vi "serial_monitor.vi"(1 "ON\nOFF":bool=TRUE caption="Init", 2 "Porta seriale":refnum<visa-resource-name>="COM3") -> ()   [LabVIEW 2014]
doc: "Lettura continua da porta seriale , INIT (true or false) della porta (9600, & bit, 1stop bit, EVEN)\nSalva su file\nFM&ADL aprile 2012"
uses:
  <vilib>/Instr/_visa.llb/VISA Configure Serial Port (Instr).vi
panel:
  out "error out":errorcluster
  out "Tutti i dati":string="MAGNETOMETRO\r\nversione Luglio 2015\r\nInizio esecuzione\r\nC9A1 D486 D53\r\n-1.69910 -1.35864 0.41638\r\n C95B D4AE D56\r\n-1.70764 -1.35376 0.41675\r\n C9AF D486 D41\r\n-1.69739 -1.35864 0.41418\r\n C997 D4B4 CED\r\n-1.70032 -1.35303 0.40393\r\n "
  in  "Baud rate":u32(ring)=9600 items=["9600"=9600, "14400"=14400, "19200"=19200, "38400"=38400, "57600"=57600, "115200"=115200]
  in  "SALVA I DATI SU FILE":bool=TRUE caption="ON\nOFF"
  out "Dati":i32[](graph)
  out "N_dati":u32
  out "lung":i32
  in  "stop":bool
  out "Number of Bytes at Serial Port":u32
  out "Dati trasmessi":string
  # "NO\nSI"
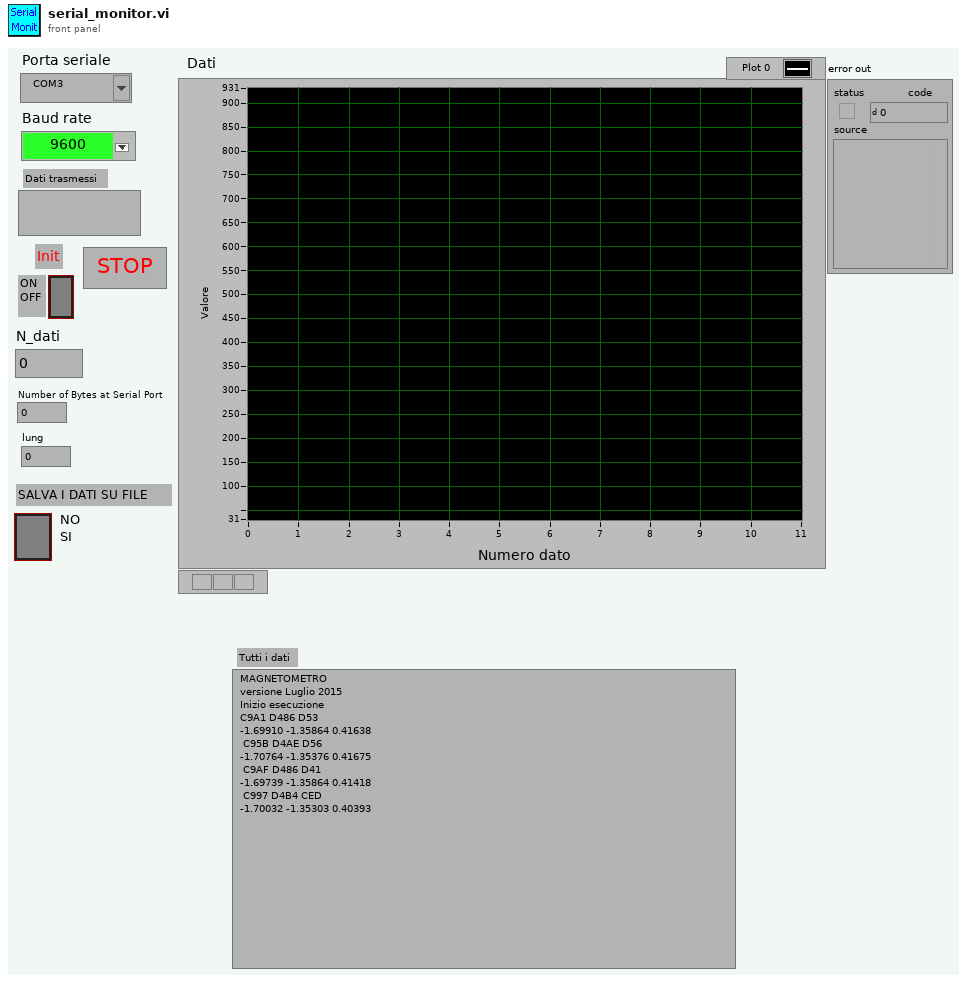
[diagram p1: front panel]
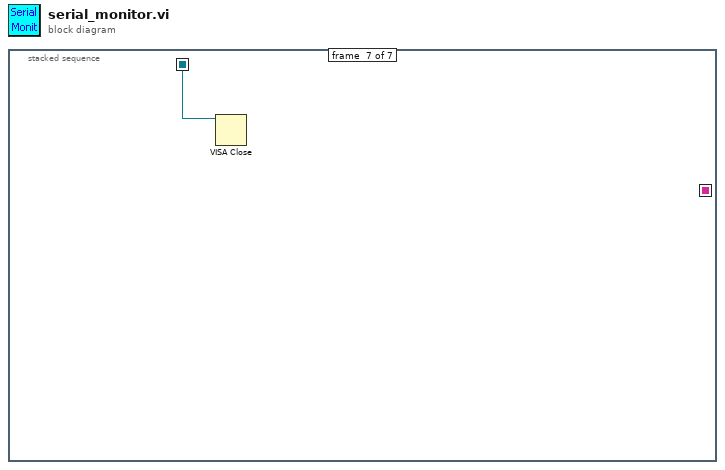
[diagram p0: block diagram]
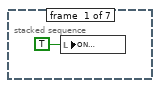
[diagram p2: hidden frame]
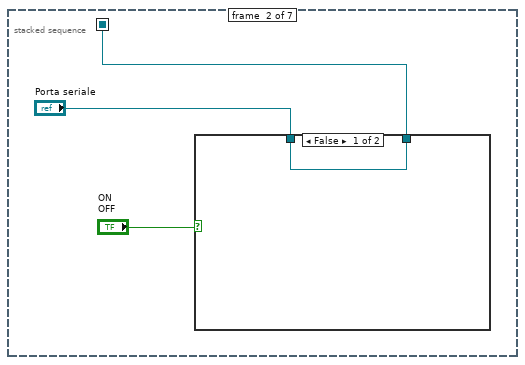
[diagram p3: hidden frame]
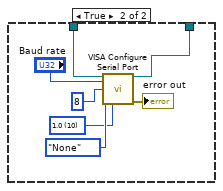
[diagram p4: hidden frame]
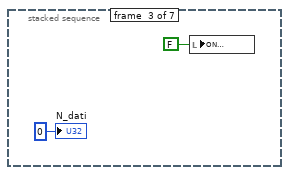
[diagram p5: hidden frame]
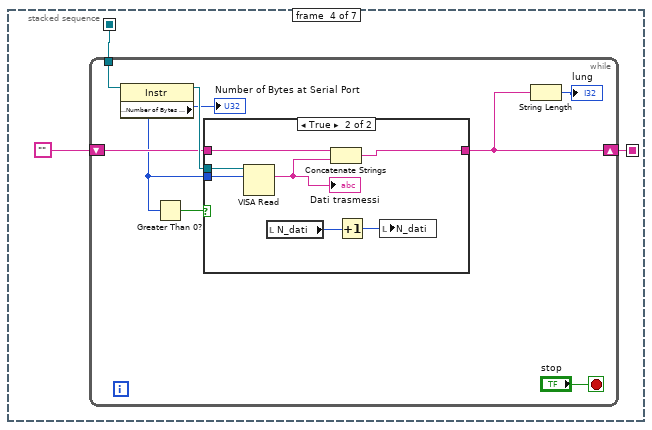
[diagram p6: hidden frame]
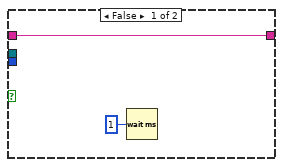
[diagram p7: hidden frame]
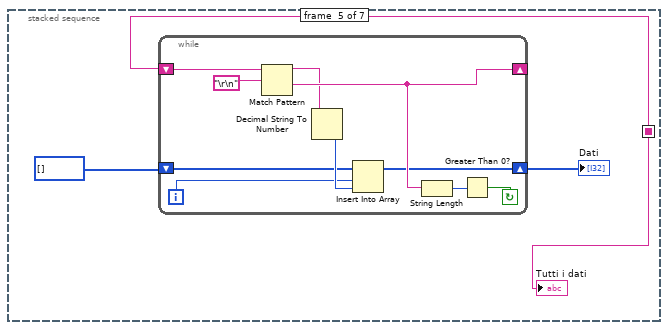
[diagram p8: hidden frame]
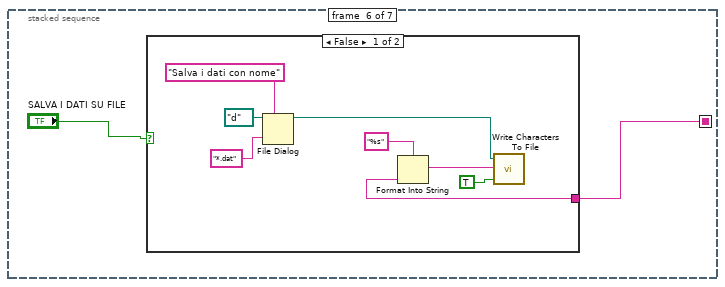
[diagram p9: hidden frame]
diagram:
  n1 = stacked-sequence {
    seq-local: [_ w2 _ _ _ _ _] -> [_ _ _ w17 _ _ w58]
    seq-local: [_ _ _ w15 _ _ _] -> [_ _ _ _ w35 w49 _]
    frame #0 {
      n2 = local write "ON\nOFF"(TRUE ("ON\nOFF")) -> ()
    }
    frame #1 {
      n3 = case shown="False" "ON\nOFF" {
        tunnel: "Porta seriale" -> [w5 w8]
        tunnel: [w5 w7] -> w2
        frame False {
        }
        frame True {
          w9 = u16 10 items=["1.0"=10, "1.5"=15, "2.0"=20] ("stop bits (10: 1 bit)")
          n4 = call-poly "VISA Configure Serial Port"("VISA resource name"=w8, "baud rate (9600)"="Baud rate", "data bits (8)"=u16 8, "parity (0:none)"=enum16{"None", "Odd", "Even", "Mark", "Space"}."None", "stop bits (10: 1 bit)"=w9) -> ("VISA resource name out"=w7:refnum<visa-resource-name>, "error out"=→"error out":errorcluster)  [unwired: 2 in, 7 out]
        }
      }
    }
    frame #2 {
      n5 = local write "ON\nOFF"(FALSE ("ON\nOFF")) -> ()
      "N_dati" <- u32 0 ("N_dati")
    }
    frame #3 {
      n6 = while {
        tunnel: w17 -> [w24]
        shift-right: [w18] -> w15
        shift-left: "" -> [w22]
        stop <- "stop" stop-if-true
        n7 = property class="Instr"(reference=w24) -> (reference out=w23:refnum<visa-resource-name>, "Serial Settings:Number of Bytes at Serial Port"=w19:u32)  [unwired: 1 in, 1 out]
        "Number of Bytes at Serial Port" <- w19
        n8 = Greater Than 0?(x=w19) -> (x > 0?=w20:bool)
        n9 = case shown="True" w20 {
          tunnel: w23 -> [_ w34]
          tunnel: w19 -> [_ w33]
          tunnel: w22 -> [w27 w32]
          tunnel: [w27 w31] -> w18
          frame False {
            n10 = Wait (ms)(milliseconds to wait=u32 1) -> ()  [unwired: 1 out]
          }
          frame True {
            n11 = VISA Read(VISA resource name=w34, byte count=w33) -> (read buffer=w30:string)  [unwired: 1 in, 3 out]
            "Dati trasmessi" <- w30
            n12 = local read "N_dati"() -> (w29:u32)
            n13 = Concatenate Strings(w32, w30) -> (w31:string)
            n14 = Increment(x=w29) -> (x+1=w28:u32)
            n15 = local write "N_dati"(w28) -> ()
          }
        }
        n16 = String Length(string=w18) -> (length=→"lung":i32)
      }
    }
    frame #4 {
      n17 = while {
        shift-right: [w39] -> w36
        shift-left: i32[] [] -> [w40]
        shift-right: [w43] -> _
        shift-left: w35 -> [w44]
        i -> [w38]
        stop <- w46 continue-if-true
        n18 = Match Pattern(string=w44, regular expression="\r\n") -> (before substring=w41:string, after substring=w43:string)  [unwired: 3 out]
        n19 = Decimal String To Number(string=w41) -> (number=w42:i32)  [unwired: 3 out]
        n20 = Insert Into Array(array=w40, index=w38, new element=w42) -> (w39:i32[])
        n21 = String Length(string=w43) -> (length=w47:i32)
        n22 = Greater Than 0?(x=w47) -> (x > 0?=w46:bool)
      }
      "Dati" <- w36
      "Tutti i dati" <- w35
    }
    frame #5 {
      n23 = case shown="False" "SALVA I DATI SU FILE" {
        tunnel: w49 -> [w57 _]
        frame False {
          n24 = File Dialog(6:"*.dat", 7:"Salva i dati con nome", 11:path "d:/" ("start path")) -> (3:w53:path)  [unwired: 1 in, 6 out]
          n25 = Format Into String(format string="%s", w57) -> (resulting string=w51:string)  [unwired: 2 in, 1 out]
          n26 = call <vilib>:"Write Characters To File.vi"("append to file? (new file:F)"=TRUE, "character string"=w51, "file path (dialog if empty)"=w53) -> ()  [unwired: 3 out]
        }
        frame True {
        }
      }
    }
    frame #6 {
      n27 = VISA Close(VISA resource name=w58) -> ()  [unwired: 1 in, 1 out]
    }
  }
